vi "CODMn测量流程.vi"(11 "控制命令":T1(ring)) -> ()   [LabVIEW 2016]
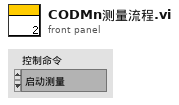
[diagram p1: front panel]
types:
  T1 = enum16{"启动测量", "标样核查", "零点核查", "跨度核查", "空白测试", "平行样测试", "加标回收", "空白校准", "标样校准", "初始化（清洗）", "停止测试", "仪器重启", "校时", "模式设置", "测量间隔设置"}
  T2 = cluster{"测量模式":enum16{"水样测量", "标样核查", "零点核查", "跨度核查", "空白测试", "加标回收", "平行样", "校零", "校标"}}
  T3 = enum16{"空闲", "水样测试", "标样核查", "零点核查", "跨度核查", "空白测试", "平行样测试", "质控样", "空白校准", "标样校准", "加标回收"}
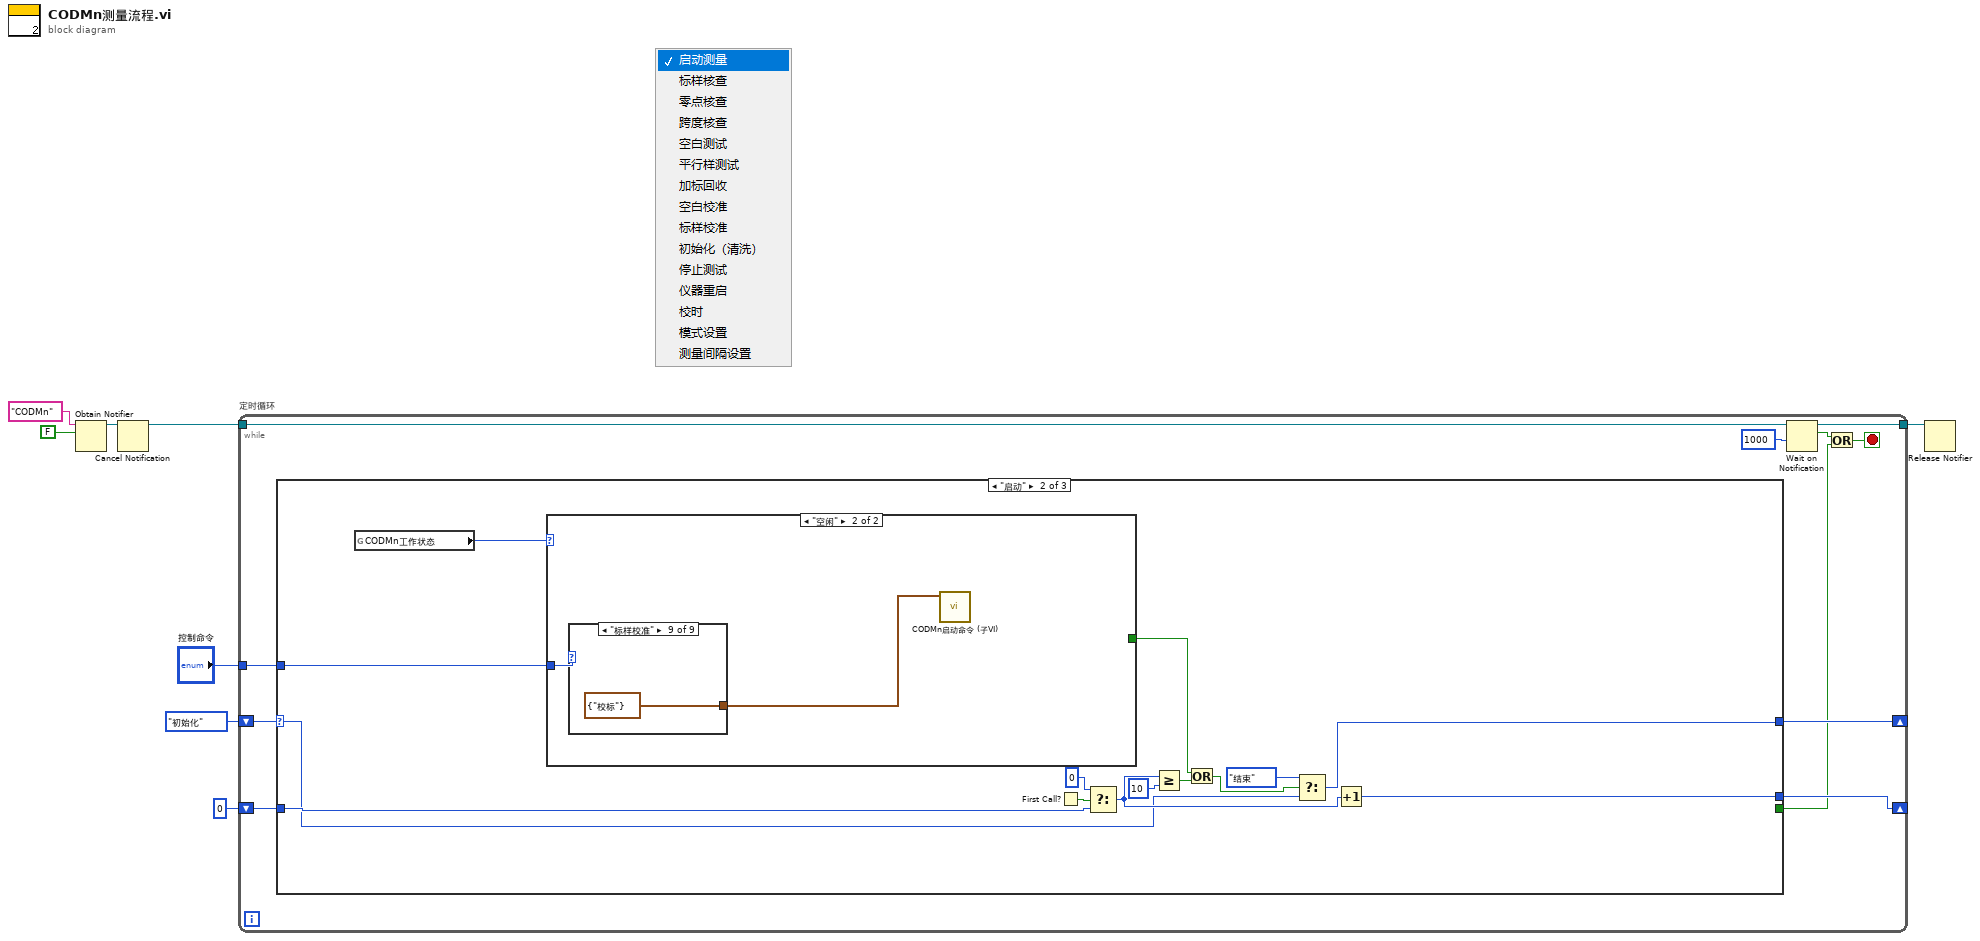
[diagram p0: block diagram]
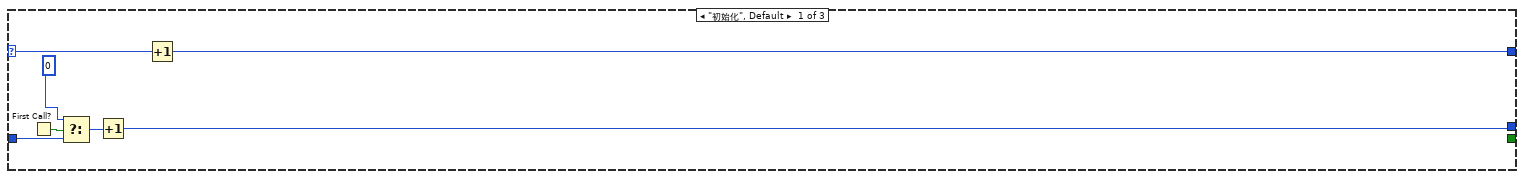
[diagram p2: hidden frame]
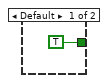
[diagram p3: hidden frame]
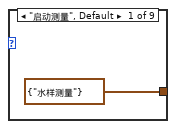
[diagram p4: hidden frame]
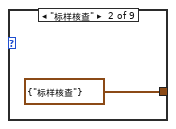
[diagram p5: hidden frame]
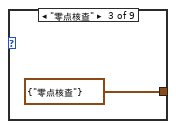
[diagram p6: hidden frame]
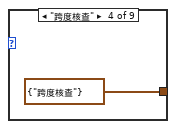
[diagram p7: hidden frame]
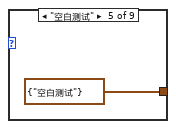
[diagram p8: hidden frame]
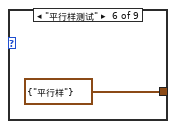
[diagram p9: hidden frame]
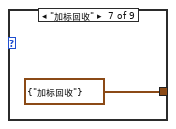
[diagram p10: hidden frame]
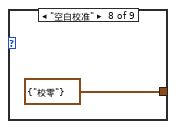
[diagram p11: hidden frame]
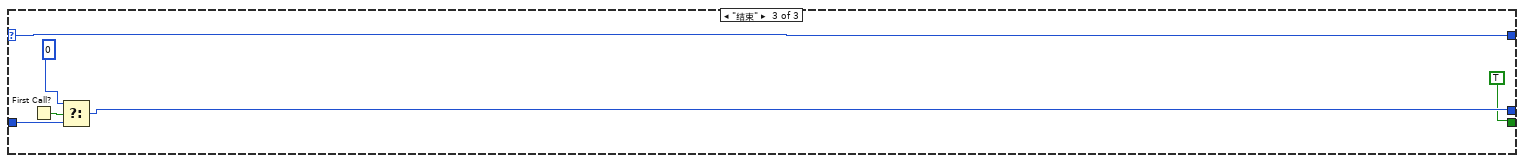
[diagram p12: hidden frame]
diagram:
  n1 = Obtain Notifier(name (unnamed)="CODMn" ("名称（未命名）"), notification data type=FALSE) -> (notifier out=w6:refnum<notifier>)  [unwired: 2 in, 2 out]
  n2 = Cancel Notification(0:w6) -> (8:w5:refnum<notifier>)  [unwired: 1 in, 2 out]
  n3 = while "定时循环" {
    tunnel: w5 -> [w19]
    tunnel: "控制命令" -> [w14]
    shift-right: [w13] -> _
    shift-left: enum16{"初始化", "启动", "结束"}."初始化" -> [w15]
    shift-right: [w11] -> _
    shift-left: 0 -> [w12]
    tunnel: [w9] -> w2
    stop <- w16 stop-if-true
    n4 = case shown="\"启动\"" w15 {
      selector: w15 -> [w26 w32 w58]
      tunnel: w14 -> [_ w40 _]
      tunnel: [w25 w33 w58] -> w13
      tunnel: w12 -> [w23 w37 w55]
      tunnel: [w20 w36 w54] -> w11
      tunnel: [_ _ TRUE] -> w10
      frame "初始化", Default {
        n5 = First Call?() -> (First Call?: T/F=w24:bool)
        n6 = Select(t=0, s=w24, f=w23) -> (s? t:f=w21:i32)
        n7 = Increment(x=w21) -> (x+1=w20:i32)
        n8 = Increment(x=w26) -> (x+1=w25:enum16{"初始化", "启动", "结束"})
      }
      frame "启动" {
        n9 = global read "COD测量模式全局.vi" "CODMn工作状态"() -> (w27:T3)
        n10 = case shown="\"空闲\"" w27 {
          tunnel: w40 -> [_ w43]
          tunnel: [TRUE _] -> w28
          frame Default {
          }
          frame "空闲" {
            n11 = case shown="\"标样校准\"" w43 {
              tunnel: [T2 {"测量模式"=enum."水样测量"} ("启动测量模式") T2 {"测量模式"=enum."标样核查"} ("启动测量模式") T2 {"测量模式"=enum."零点核查"} ("启动测量模式") T2 {"测量模式"=enum."跨度核查"} ("启动测量模式") T2 {"测量模式"=enum."空白测试"} ("启动测量模式") T2 {"测量模式"=enum."平行样"} ("启动测量模式") T2 {"测量模式"=enum."加标回收"} ("启动测量模式") T2 {"测量模式"=enum."校零"} ("启动测量模式") T2 {"测量模式"=enum."校标"} ("启动测量模式")] -> w42
              frame "启动测量", Default {
              }
              frame "标样核查" {
              }
              frame "零点核查" {
              }
              frame "跨度核查" {
              }
              frame "空白测试" {
              }
              frame "平行样测试" {
              }
              frame "加标回收" {
              }
              frame "空白校准" {
              }
              frame "标样校准" {
              }
            }
            n12 = call "CODMn启动命令 (子VI).vi"("启动测量模式"=w42) -> ()  [unwired: 11 in]
          }
        }
        n13 = First Call?() -> (First Call?: T/F=w39:bool)
        n14 = Select(t=0, s=w39, f=w37) -> (s? t:f=w35:i32)
        n15 = Greater Or Equal?(x=w35, y=10) -> (x >= y?=w31:bool)
        n16 = Or(x=w28, y=w31) -> (x .or. y?=w29:bool)
        n17 = Select(t=enum16{"初始化", "启动", "结束"}."结束", s=w29, f=w32) -> (s? t:f=w33:enum16{"初始化", "启动", "结束"})
        n18 = Increment(x=w35) -> (x+1=w36:i32)
      }
      frame "结束" {
        n19 = First Call?() -> (First Call?: T/F=w57:bool)
        n20 = Select(t=0, s=w57, f=w55) -> (s? t:f=w54:i32)
      }
    }
    n21 = Wait on Notification(notifier=w19, timeout in ms (-1)=1000 ("超时毫秒(-1)")) -> (notifier out=w9:refnum<notifier>, notification=w17:bool)  [unwired: 2 in, 2 out]
    n22 = Or(x=w17, y=w10) -> (x .or. y?=w16:bool)
  }
  n23 = Release Notifier(notifier=w2) -> ()  [unwired: 2 in, 3 out]
